vi "Pressure_Tapped_Cube.vi"(3 "Mode":T5, 5 "Traverse line In":T2 {"Carrier_2 Q (l/min)" format="%#.2f"; "Row Duration (mins)" format="%#.1f"; "Row No" min=0; "Trace Gas Concentration (%)" min=0.0 format="%#_4f"; "Carrier_1 Q (l/min)" format="%#.2f"; "Tunnel Speed" format="%#.2f"; "Start X" format="%#.2f"; "Start Y" format="%#.2f"; "Start Z" format="%#.2f"; "End X" format="%#.2f"; "End Y" format="%#.2f"; "End Z" format="%#.2f"; "Averaging time (min)" min=0.0 format="%#.2f"}) -> (0 "Error Message":string, 1 "Status":T1, 2 "Traverse line Out":T2 {"Carrier_2 Q (l/min)" format="%#.2f"; "Row Duration (mins)" format="%#.1f"; "Row No" min=0; "Trace Gas Concentration (%)" min=0.0 format="%#_4f"; "Carrier_1 Q (l/min)" format="%#.2f"; "Tunnel Speed" format="%#.2f"; "Start X" format="%#.2f"; "Start Y" format="%#.2f"; "Start Z" format="%#.2f"; "End X" format="%#.2f"; "End Y" format="%#.2f"; "End Z" format="%#.2f"; "Averaging time (min)" min=0.0 format="%#.2f"})   [LabVIEW 2014]
uses:
  Gen Trav/Traverse_cluster.ctl
  Gen Trav/Spacing.ctl
  Controls/Multi_run_mode.ctl
  Controls/User_Specific_mode.ctl
  Gen Trav/Multi_Run_Status.ctl
  Gen Trav/Trav_mode.ctl
  Controls/Setup.ctl
  Controls/Save_Data.ctl
  <vilib>/Analysis/baseanly.llb/Mean (DBL).vi
  Globals/Meas_global.vi
  <vilib>/Analysis/NI_AALBase.lvlib
panel:
  out "XY Graph":cluster{dbl[], dbl[]}(graph)
  out "Measurement No":i32
  in  "stop":bool
  # "X           Y            Z"
  # "Start"
  # "End"
  # "X           Y            Z"
  # "Start"
  # "End"
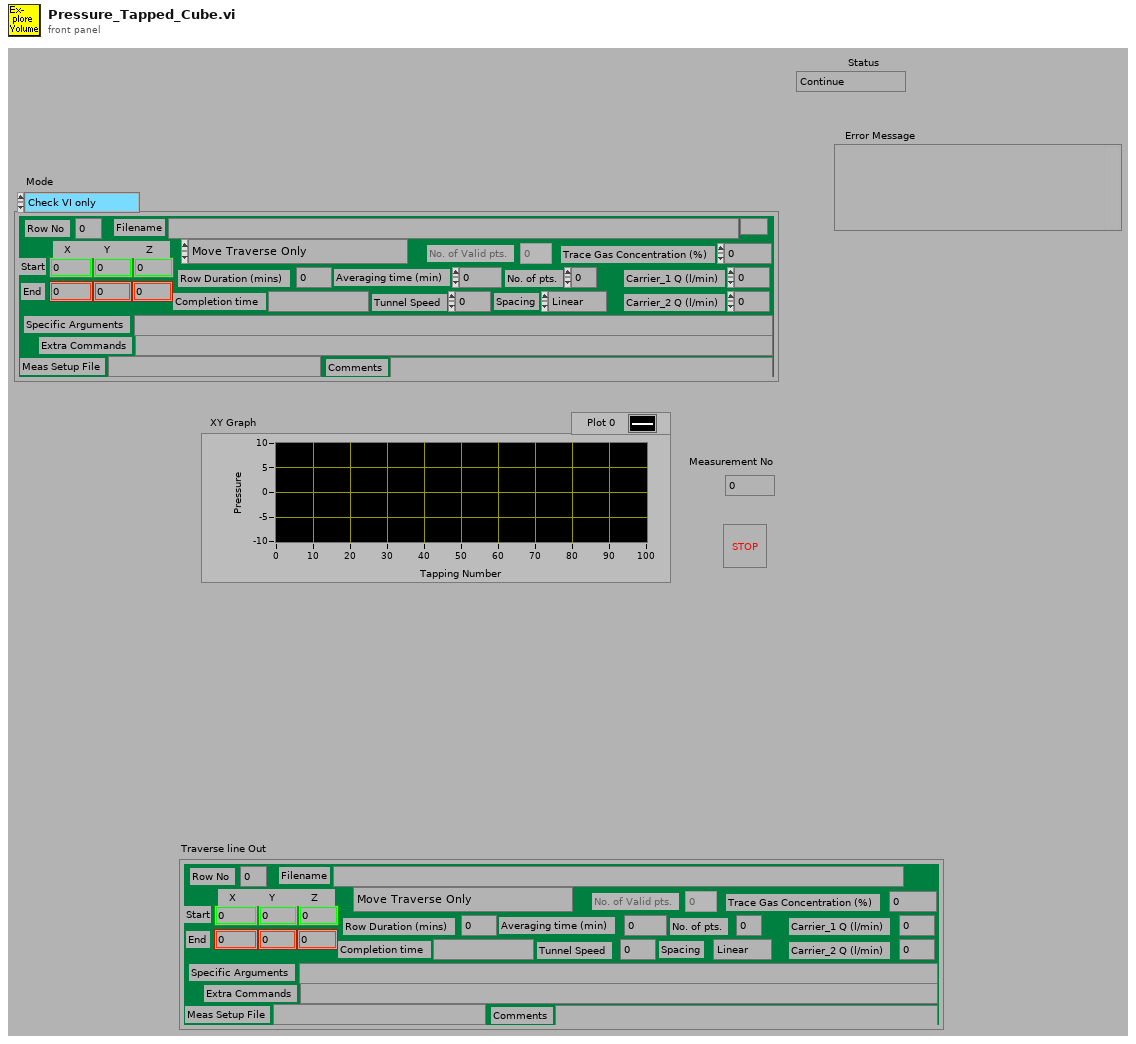
[diagram p1: front panel]
types:
  T1 = typedef "Multi_Run_Status.ctl" = enum16{"Continue", "Jump to Next Point", "Jump to Next Row", "Jump To Fall Back", "Terminate Run"}
  T2 = typedef "Traverse_cluster.ctl" = cluster{"Start X":sgl, "Start Y":sgl, "Start Z":sgl, "End X":sgl, "End Y":sgl, "End Z":sgl, "No. of pts.":i32, "Spacing":T3, "Filename":path, "Tunnel Speed":dbl, "Averaging time (min)":dbl, "Extra Commands":string, "Carrier_1 Q (l/min)":dbl, "Carrier_2 Q (l/min)":dbl, "Trace Gas Concentration (%)":dbl, "Specific Arguments":string, "Comments":string, "Row No":i32, "Row Type Selector":T4, "Completion time":string, "Row Duration (mins)":dbl, "No. of Valid pts.":i32, "Meas Setup File":string}
  T3 = typedef "Spacing.ctl" = enum16{"Linear", "Log", "Gauss", "Specified", "N/A"}
  T4 = typedef "Multi_run_mode.ctl" = enum16{"Move Traverse Only", "Set Tunnel Speed Only", "Set Source Only", "Set Measurement Conditions", "Single Measurement", "Vertical Profile", "Lateral Profile", "Longitudinal Profile", "Explore Volume", "Multi-Axis Profile", "Auto Calibrate", "Meas Fast FID Bkgnd", "Check Beam Power", "Scanning Valve Measurement", "Run VI Named:", "Set ADAM Ch", "Wait (minutes)", "Send Message", "Synchronize With:", "Fall Back to this Row", "Turn Off Row Repeating", "Blank Row", "Traverse 3D Volume"}
  T5 = typedef "User_Specific_mode.ctl" = enum16{"Check VI only", "Run VI"}
  T6 = typedef "Trav_mode.ctl" = enum16{"Move traverse", "Read traverse position", "Teach Position"}
  T7 = typedef "Save_Data.ctl" = enum16{"Save No Data", "Save Data"}
  T8 = typedef "Setup.ctl" = enum16{"Run Program", "Show Setup", "Save Current Setup", "Setup Front Panel"}
  T9 = typedef "Status_Cluster.ctl" = cluster{"Status":T1, "Error Type":string, "Error Description":string}
  T10 = typedef "Analysis_info_cluster.ctl" = cluster{"Colour":u32, "Inst type":T11, "Inst name":string, "Symbol":string, "Code name":string, "Extra Info":string, "Inst Array":T12, "Extra Titles":string[], "Extra Values":string[], "U":dbl, "u^2":dbl, "u^3":dbl, "u^4":dbl, "Skew_u":dbl, "Kurt_u":dbl, "Sd Error in Mean":dbl, "% u'/U":dbl, "X":dbl, "Y":dbl, "Z":dbl, "Timescale integral to 25%":dbl, "Sd Error in Variance":dbl, "Calib File":path, "Calib Constants":dbl[], "Output Position":bool, "Full Stats":bool, "Av Sampling Rate":dbl, "Av No of Samples":dbl, "Total Meas Time (s)":dbl, "ADAM Ch Name":string}
  T11 = typedef "Inst_type.ctl" = enum16{"Propeller anemometer", "Raw voltage", "Pressure Transducer", "Pitot-static tube", "Preston tube", "Hot wire", "Cross wire 1", "Cross wire 2", "Generic Linear", "Generic Polynomial", "Generic BackPoly", "Fast FID", "Thermocouple", "Cold wire", "Pulsed Wire", "LDA Vel", "LDA Tran time", "LDA Arr time", "Microphone"}
  T12 = typedef "Instrument_Array.ctl" = enum16{"PWA", "LDA", "Analogue"}
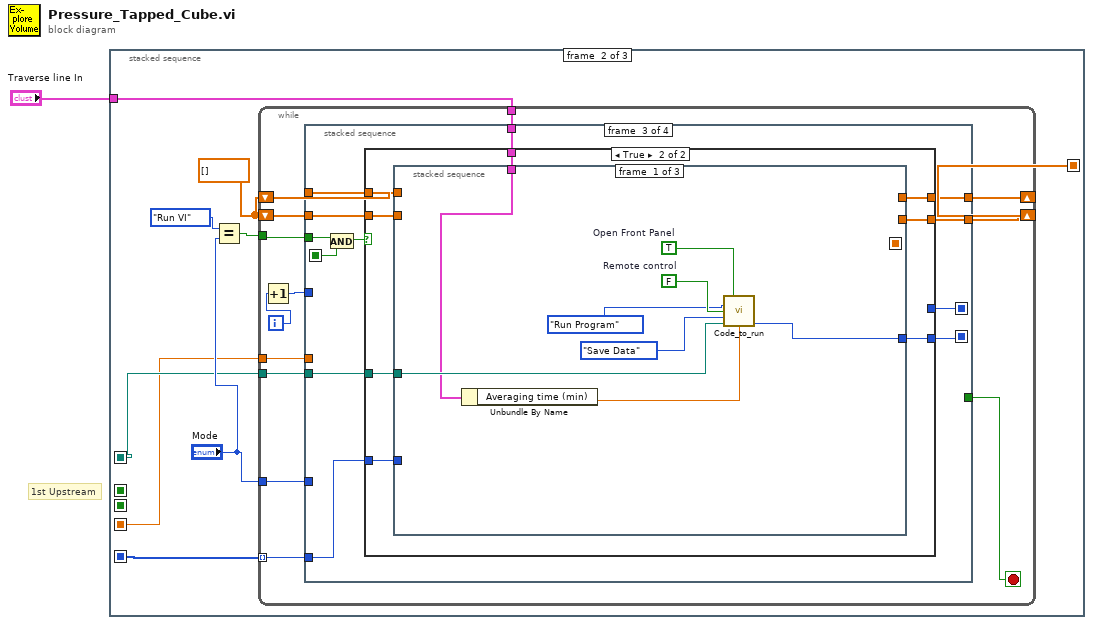
[diagram p0: block diagram]
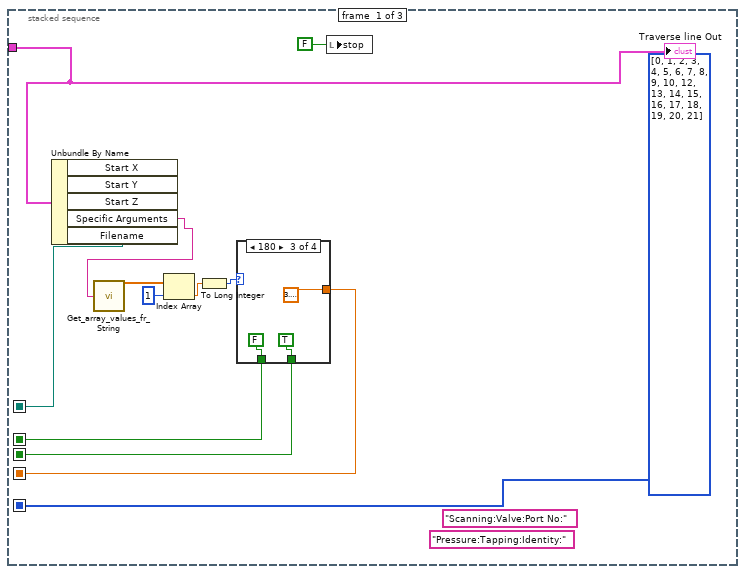
[diagram p2: hidden frame]
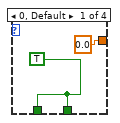
[diagram p3: hidden frame]
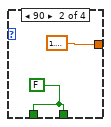
[diagram p4: hidden frame]
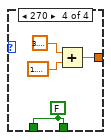
[diagram p5: hidden frame]
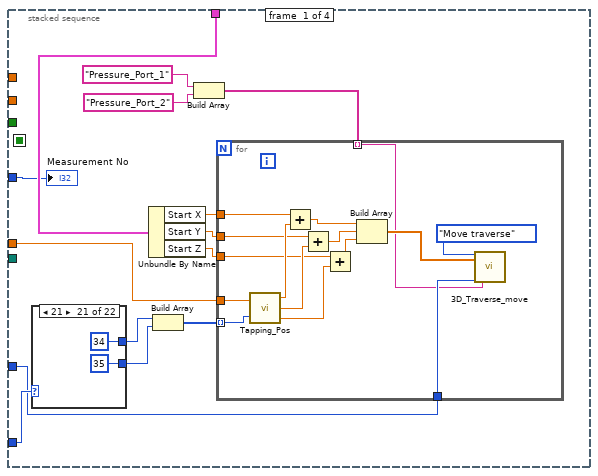
[diagram p6: hidden frame]
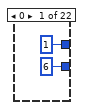
[diagram p7: hidden frame]
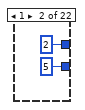
[diagram p8: hidden frame]
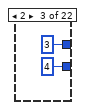
[diagram p9: hidden frame]
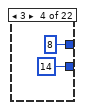
[diagram p10: hidden frame]
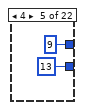
[diagram p11: hidden frame]
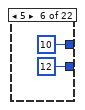
[diagram p12: hidden frame]
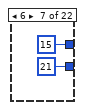
[diagram p13: hidden frame]
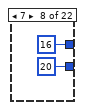
[diagram p14: hidden frame]
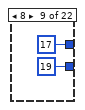
[diagram p15: hidden frame]
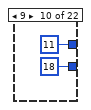
[diagram p16: hidden frame]
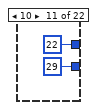
[diagram p17: hidden frame]
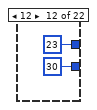
[diagram p18: hidden frame]
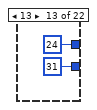
[diagram p19: hidden frame]
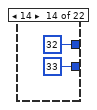
[diagram p20: hidden frame]
diagram:
  # "1st Upstream"
  n1 = stacked-sequence {
    seq-local: [w2 _ _] -> [_ w30 _]
    seq-local: [_ w29 _] -> [_ _ w228]
    seq-local: [w6 _ _] -> [_ _ w223]
    seq-local: [w4 _ _] -> [_ w26 _]
    seq-local: [w5 _ _] -> [_ _ w213]
    seq-local: [i32[] [0, 1, 2, 3, 4, 5, 6, 7, 8, 9, 10, 12, 13, 14, 15, 16, 17, 18, 19, 20, 21] _ _] -> [_ w25 _]
    tunnel: "Traverse line In" -> [w13 w27 _]
    frame #0 {
      (unwired) "Pressure:Tapping:Identity:"
      (unwired) "Scanning:Valve:Port No:"
      n2 = Unbundle By Name(w13) -> ("Specific Arguments"=w12:string, "Filename"=w2:path)  [unwired: 3 out]
      n3 = call "Get_array_values_fr_String.vi"("String Value"=w12) -> ("Numeric Array"=w10:dbl[])  [unwired: 1 out]
      n4 = Index Array(array=w10, index=1) -> (element=w8:dbl)
      n5 = To Long Integer(number=w8) -> (32bit integer=w7:i32)
      n6 = case shown="180" w7 {
        tunnel: [0.0 1.5707963267948966 3.141592653589793 w22] -> w4
        tunnel: [w14 w16 FALSE w21] -> w6
        tunnel: [w14 w16 TRUE w21] -> w5
        frame 0, Default {
          w14 = TRUE
        }
        frame 90 {
          w16 = FALSE
        }
        frame 180 {
        }
        frame 270 {
          w21 = FALSE
          n7 = Add(x=3.141592653589793, y=1.5707963267948966) -> (x+y=w22:dbl)
        }
      }
      n8 = local write "stop"(FALSE ("stop")) -> ()
      "Traverse line Out" <- w13
    }
    frame #1 {
      w28 = dbl[] []
      n9 = Equal?(x=User_Specific_mode."Run VI" ("Mode"), y="Mode") -> (x = y?=w31:bool)
      n10 = while {
        tunnel: "Mode" -> [w41]
        tunnel: w31 -> [w37]
        tunnel: w30 -> [w46]
        shift-right: [w44] -> w29
        shift-left: w28 -> [w45]
        shift-right: [w42] -> _
        shift-left: w28 -> [w43]
        tunnel: w27 -> [w40]
        tunnel: w26 -> [w39]
        tunnel: w25 -> [w34] mode=indexing
        i -> [w36]
        stop <- w38 stop-if-true
        n11 = Increment(x=w36) -> (x+1=w35:i32)
        n12 = stacked-sequence {
          seq-local: [_ w123 _ _] -> [_ _ w150 _]
          seq-local: [_ w122 _ _] -> [_ _ w151 _]
          seq-local: [_ _ w152 _] -> [_ _ _ w205]
          tunnel: w46 -> [_ _ w158 _]
          tunnel: w45 -> [_ _ w157 _]
          tunnel: [_ _ w156 _] -> w44
          tunnel: w43 -> [_ _ w155 _]
          tunnel: [_ _ w154 _] -> w42
          tunnel: w41 -> [w52 w126 _ _]
          tunnel: w40 -> [w60 w133 w153 _]
          tunnel: w35 -> [w54 _ _ w208]
          tunnel: w39 -> [w59 _ _ _]
          tunnel: [_ _ _ w206] -> w38
          tunnel: w37 -> [_ _ w149 _]
          tunnel: w34 -> [w53 w121 w147 _]
          frame #0 {
            n13 = case shown="21" w53 {
              tunnel: [1 2 3 8 9 10 15 16 17 11 22 23 24 32 36 37 39 41 26 28 34 -1] -> w58
              tunnel: [6 5 4 14 13 12 21 20 19 18 29 30 31 33 25 38 40 42 27 7 35 -1] -> w57
              frame 0 {
              }
              frame 1 {
              }
              frame 2 {
              }
              frame 3 {
              }
              frame 4 {
              }
              frame 5 {
              }
              frame 6 {
              }
              frame 7 {
              }
              frame 8 {
              }
              frame 9 {
              }
              frame 10 {
              }
              frame 12 {
              }
              frame 13 {
              }
              frame 14 {
              }
              frame 15 {
              }
              frame 16 {
              }
              frame 17 {
              }
              frame 18 {
              }
              frame 19 {
              }
              frame 20 {
              }
              frame 21 {
              }
              frame 22, Default {
              }
            }
            n14 = Unbundle By Name(w60) -> ("Start X"=w55:sgl, "Start Y"=w47:sgl, "Start Z"=w48:sgl)
            n15 = Build Array(w58, w57) -> (w56:i32[])
            n16 = Build Array("Pressure_Port_1", "Pressure_Port_2") -> (w49:string[])
            n17 = for {
              tunnel: w59 -> [w119]
              tunnel: w56 -> [w118] mode=indexing
              tunnel: w55 -> [w117]
              tunnel: w52 -> [w112]
              tunnel: w49 -> [w111] mode=indexing
              tunnel: w48 -> [w106]
              tunnel: w47 -> [w105]
              n18 = call "Tapping_Pos.vi"("Orientation"=w119, "Tapping Number"=w118) -> ("X"=w116:sgl, "Y"=w107:sgl, "Z"=w108:sgl)
              n19 = Add(x=w117, y=w116) -> (x+y=w115:sgl)
              n20 = Add(x=w105, y=w107) -> (x+y=w109:sgl)
              n21 = Add(x=w106, y=w108) -> (x+y=w110:sgl)
              n22 = Build Array(w115, w109, w110) -> (w114:sgl[])
              n23 = call "3D_Traverse_move.vi"("Mode"=Trav_mode."Move traverse", "Position"=w114, "Simulate/Run"=w112, "Traverse name"=w111) -> ()  [unwired: 13 in, 3 out]
            }
            "Measurement No" <- w54
          }
          frame #1 {
            w120 = sgl nan ("Start X")
            n24 = case shown="\"Check VI only\", Default" w126 {
              tunnel: w121 -> [_ w137]
              tunnel: ["" w136] -> w127
              frame "Check VI only", Default {
              }
              frame "Run VI" {
                n25 = call "ScaniValve_client.vi"("Port Number"=w137) -> ("Error String"=w136:string)  [unwired: 2 out]
              }
            }
            n26 = Empty String/Path?(string/path=w127) -> (empty?=w130:bool)
            n27 = Not(x=w130) -> (.not. x?=w129:bool)
            n28 = Bundle By Name(cluster=w133, "Row Type Selector"=Multi_run_mode."Set Measurement Conditions", "Start X"=w120, "Start Y"=w120, "Start Z"=w120) -> (w131:T2)
            n29 = call "Set_Measurement_Conditions.vi"("Simulate/Run"=w126, "Currently on Point"=1, "Traverse line"=w131) -> ("Status Cluster"=w128:T9)  [unwired: 2 out]
            n30 = case shown="True" w129 {
              tunnel: w128 -> [w138 w146]
              tunnel: [w138 w143] -> w124
              tunnel: w127 -> [_ w140]
              tunnel: w121 -> [_ w139]
              frame False {
              }
              frame True {
                n31 = Format Into String(format string=" For Port No %d." ("Format String"), initial string=w140, w139) -> (resulting string=w141:string)  [unwired: 1 in, 1 out]
                n32 = Bundle By Name(cluster=w146, "Status"=Multi_Run_Status."Jump to Next Point", "Error Type"="Scanning Valve Error" ("t"), "Error Description"=w141) -> (w143:T9)
              }
            }
            n33 = Unbundle By Name(w124) -> ("Status"=w122:T1)
            n34 = Equal?(x=Multi_Run_Status."Continue" ("Status"), y=w122) -> (x = y?=w123:bool)
            n35 = call "Prog_Status_Handler.vi"("Status Cluster"=w124, "Simulate/Run"=w126) -> ()  [unwired: 2 out]
          }
          frame #2 {
            n36 = And(x=w149, y=w150) -> (x .and. y?=w148:bool)
            n37 = case shown="True" w148 {
              tunnel: [w159 w169] -> w152
              tunnel: w158 -> [_ w168]
              tunnel: w157 -> [w161 w167]
              tunnel: [w161 w166] -> w156
              tunnel: w155 -> [w160 w165]
              tunnel: [w160 w164] -> w154
              tunnel: w153 -> [_ w163]
              tunnel: w147 -> [_ w162]
              tunnel: w151 -> [w159 _]
              frame False {
                (unwired) FALSE ("stop")
              }
              frame True {
                n38 = stacked-sequence {
                  seq-local: [_ w180 _] -> [_ _ w196]
                  tunnel: [w172 _ _] -> w169
                  tunnel: w168 -> [w171 _ _]
                  tunnel: w167 -> [_ w181 _]
                  tunnel: [_ w180 _] -> w166
                  tunnel: w165 -> [_ _ w201]
                  tunnel: [_ _ w199] -> w164
                  tunnel: w163 -> [w170 _ _]
                  tunnel: w162 -> [_ _ w194]
                  frame #0 {
                    w175 = TRUE  # Open Front Panel
                    w177 = FALSE  # Remote control
                    n39 = Unbundle By Name(w170) -> ("Averaging time (min)"=w176:dbl)
                    n40 = call "Code_to_run.vi"("Open Front Panel"=w175, "setup"=Setup."Run Program", "Remote control"=w177, "File"=Save_Data."Save Data", "Results Filename"=w171, "Averaging time (min)"=w176) -> ("Status"=w172:T1)  [unwired: 5 in, 4 out]
                  }
                  frame #1 {
                    n41 = global read "Meas_global.vi" "Analysis Info cluster"() -> (w179:T10[])
                    n42 = Array Size(array=w179) -> (size(s)=w178:i32)
                    n43 = while {
                      tunnel: w179 -> [w193] mode=indexing
                      tunnel: [w191] -> _ mode=indexing
                      tunnel: [w192] -> w182
                      tunnel: w178 -> [w188]
                      i -> [w189]
                      stop <- w183 continue-if-true
                      n44 = Decrement(x=w188) -> (x-1=w187:i32)
                      n45 = Unbundle By Name(w193) -> ("Inst name"=w191:string, "U"=w192:dbl)
                      n46 = Match Pattern(string=w191, regular expression="Mano") -> (offset past match=w186:i32)  [unwired: 4 out]
                      n47 = Less?(x=w189, y=w187) -> (x < y?=w184:bool)
                      n48 = Less Than 0?(x=w186) -> (x < 0?=w185:bool)
                      n49 = And(x=w185, y=w184) -> (x .and. y?=w183:bool)
                    }
                    n50 = Build Array (concatenate)(w181, w182) -> (w180:dbl[])
                  }
                  frame #2 {
                    n51 = Build Array (concatenate)(w201, w194) -> (w199:dbl[])
                    n52 = call "Sort_Array_Indicies.vi"("unsorted array"=w199) -> ("sorted array"=w198:dbl[], "Sort Index"=w197:i32[])
                    n53 = for {
                      tunnel: w197 -> [w204] mode=indexing
                      tunnel: w196 -> [w203]
                      tunnel: [w202] -> w195 mode=indexing
                      n54 = Index Array(array=w203, index=w204) -> (element=w202:dbl)
                    }
                    n55 = Bundle("sorted array"=w198, w195) -> (→"XY Graph":cluster{"sorted array":dbl[], dbl[]})  [unwired: 1 out]
                  }
                }
              }
            }
          }
          frame #3 {
            n56 = Greater?(x=w205, y=Multi_Run_Status."Jump to Next Point" ("Status")) -> (0:w211:bool)
            n57 = Greater Or Equal?(x=w208, y=21.0) -> (x >= y?=w210:bool)
            n58 = Compound Arithmetic op=OR("stop", w211, w210) -> (w206:bool)
            "Status" <- w205
          }
        }
      }
    }
    frame #2 {
      n59 = Split 1D Array(array=w228, index=21) -> (first subarray=w226:dbl[], second subarray=w222:dbl[])
      n60 = Array Size(array=w222) -> (size(s)=w221:i32)
      n61 = call-poly <vilib>:"Mean.vi"("X"=w226) -> ("mean"=w225:dbl)  [unwired: 1 out]
      n62 = call-poly <vilib>:"Mean.vi"("X"=w222) -> ("mean"=w224:dbl)  [unwired: 1 out]
      n63 = Greater?(x=w221, y=19) -> (0:w214:bool)
      n64 = case shown="False" w223 {
        tunnel: w225 -> [w231 w234]
        tunnel: w224 -> [w230 w233]
        tunnel: [w229 w232] -> w219
        frame False {
          n65 = Greater?(x=w231, y=w230) -> (0:w229:bool)
        }
        frame True {
          n66 = Less?(x=w234, y=w233) -> (x < y?=w232:bool)
        }
      }
      n67 = Compound Arithmetic op=AND(w219, w214, w213) -> (w218:bool)
      n68 = Select(t="The Pressures on the upstream face are lower than the downstream face.\nMaybe you have incorrectly entered the orientation of the cube via the second specific argument.", s=w218, f="") -> (s? t:f=→"Error Message":string)
    }
  }
